vi "Mapping v10.0.0.vi"(5 "Simulate Spectra":bool, 7 "Simulate Drive":bool, 11 "Input Parameters":T7={"CCD3000 Connection"={"Comm Interface"=1, "BUS"=0, "Address"=5, "Com Port"=1}, "Drive Connection Settings"={"Objective GPIB-Port"=4, "Stage GPIB-Port"=4, "Drive Selector"=0, "Drive Velocity (V/s)"=5.0}, "ITC503 Current Values"={"ITC503 Heater"=0.0, "ITC503 Temperature"=0.0, "ITC503 P"=0.0, "ITC503 I"=0.0, "ITC503 D"=0.0, "ITC503 Setpoint"=0.0, "ITC503 Gradient"=0.0, "ITC503 Heater Auto"=FALSE, "ITC503 PID Auto"=FALSE}, "Wavelengths (nm)"=[], "Drive Current Values"={"Voltages"={"Drive X Voltage"=0.0, "Drive Y Voltage"=0.0, "Drive Z Voltage"=0.0}, "Position"={"Drive X Position"=0.0, "Drive Y Position"=0.0, "Drive Z Position"=0.0}}, "iHR Current Values"={"iHR 550 Front Entrance"=0.0, "iHR550 Side Exit"=0.0, "iHR550 Wavelength"=897.9988, "iHR550 Exit Mirror"=2, "iHR550 Grating"="1", "Grating Index"=1}, "Spectra Settings"={"Integration Time"=1.0, "Repetitions"=1, "Mapping Spectra"=TRUE}, "CCD3500 Temperature"=0.0} {"CCD3500 Temperature" min=10.0 max=160.0 step=0.1 format="%.1f"; "Spectra Settings"."Repetitions" min=1 max=100 step=1; "Spectra Settings"."Integration Time" min=0.5 max=6000.0 step=1.0 format="%.1f"; "iHR Current Values"."iHR550 Exit Mirror" items=["EntranceMirror", "ExitMirror", "Front", "Side"]; "Drive Current Values"."Position"."Drive Z Position" min=-273.0 max=300000.0 step=0.0001 format="%.1f"; "Drive Current Values"."Position"."Drive Y Position" min=-273.0 max=300000.0 step=0.0001 format="%.1f"; "Drive Current Values"."Position"."Drive X Position" min=-273.0 max=300000.0 step=0.0001 format="%.1f"; "Drive Current Values"."Voltages"."Drive Z Voltage" min=-273.0 max=300000.0 step=0.0001 format="%.1f"; "Drive Current Values"."Voltages"."Drive Y Voltage" min=-273.0 max=300000.0 step=0.0001 format="%.1f"; "Drive Current Values"."Voltages"."Drive X Voltage" min=-273.0 max=300000.0 step=0.0001 format="%.1f"; "ITC503 Current Values"."ITC503 Gradient" format="%.2f"; "ITC503 Current Values"."ITC503 Setpoint" min=-273.0 max=300000.0 step=0.0001 format="%.1f"; "ITC503 Current Values"."ITC503 I" format="%_1f"; "ITC503 Current Values"."ITC503 P" format="%_1f"; "ITC503 Current Values"."ITC503 Temperature" min=0.0 max=1645.0 step=1e-05 format="%.2f"; "ITC503 Current Values"."ITC503 Heater" min=0.0 max=100.0 step=0.01 scale=0.0..100.0; "Drive Connection Settings"."Drive Velocity (V/s)" min=10.0 max=160.0 step=0.1 format="%.1f"; "Drive Connection Settings"."Drive Selector" items=["Obj.", "Stage"]; "Drive Connection Settings"."Stage GPIB-Port" min=1 max=20 step=1 format="%#.0f"; "Drive Connection Settings"."Objective GPIB-Port" min=1 max=20 step=1 format="%#.0f"; "CCD3000 Connection"."Comm Interface" items=["RS 232", "GPIB"]}) -> ()   [LabVIEW 2010]
uses:
  ESA-C/TypeDefs/ESA-C Connection Settings.ctl
  TypeDefs/Mapping Spectra Params.ctl
  TypeDefs/Mapping Drive Params.ctl
  ESA-C/TypeDefs/ESA-C Set Positions.ctl
  ESA-C/TypeDefs/ESA-C Current Values.ctl
  iHR550/TypeDefs/iHR Current Values.ctl
  ITC503/TypeDefs/ITC503 Current Values.ctl
  drivers/Horiba Spectrum One 3000V/Lib/CCD_command.llb/Comm Params.ctl
  <vilib>/Utility/miscctls.llb/LVPointTypeDef.ctl
panel:
  in  "CCD3000 Current Rep.":string="0/0"
  in  "CCD3500V Connection":T8={"Comm Interface"=1, "BUS"=0, "Address"=5, "Com Port"=0}
  out "Live Data":dbl[][](array[numeric])
  in  "ITC503 Current Values":T3 {"ITC503 Gradient" format="%.2f"; "ITC503 Setpoint" min=-273.0 max=300000.0 step=0.0001 format="%.1f"; "ITC503 I" format="%_1f"; "ITC503 P" format="%_1f"; "ITC503 Temperature" min=0.0 max=1645.0 step=1e-05 format="%.2f"; "ITC503 Heater" min=0.0 max=100.0 step=0.01 scale=0.0..100.0}
  in  "iHR Current Values":T5={"iHR 550 Front Entrance"=0.0, "iHR550 Side Exit"=0.0, "iHR550 Wavelength"=897.9988, "iHR550 Exit Mirror"=2, "iHR550 Grating"="1", "Grating Index"=1} {"iHR550 Exit Mirror" items=["EntranceMirror", "ExitMirror", "Front", "Side"]}
  in  "CCD3500 Temperature":dbl caption="Temp. (°C)" min=10.0 max=160.0 step=0.1 format="%.1f"
  in  "Wavelengths (nm)":dbl[](array[numeric])
  in  "Spectra Params":T6={"Integration Time"=10.0, "Repetitions"=10, "Mapping Spectra"=TRUE} {"Repetitions" min=1 max=100 step=1; "Integration Time" min=0.5 max=6000.0 step=1.0 format="%.1f"}
  in  "Drive Settings":T2={"Objective GPIB-Port"=4, "Stage GPIB-Port"=4, "Drive Selector"=0, "Drive Velocity (V/s)"=5.0} {"Drive Velocity (V/s)" min=10.0 max=160.0 step=0.1 format="%.1f"; "Drive Selector" items=["Obj.", "Stage"]; "Stage GPIB-Port" min=1 max=20 step=1 format="%#.0f"; "Objective GPIB-Port" min=1 max=20 step=1 format="%#.0f"}
  out "Current Position":T4 {"Position"."Drive Z Position" min=-273.0 max=300000.0 step=0.0001 format="%.1f"; "Position"."Drive Y Position" min=-273.0 max=300000.0 step=0.0001 format="%.1f"; "Position"."Drive X Position" min=-273.0 max=300000.0 step=0.0001 format="%.1f"; "Voltages"."Drive Z Voltage" min=-273.0 max=300000.0 step=0.0001 format="%.1f"; "Voltages"."Drive Y Voltage" min=-273.0 max=300000.0 step=0.0001 format="%.1f"; "Voltages"."Drive X Voltage" min=-273.0 max=300000.0 step=0.0001 format="%.1f"}
  out "Target Position":T9={"Drive X Set"=10.0, "Drive Y Set"=10.0, "Drive Z Set"=10.0} {"Drive X Set" min=10.0 max=160.0 step=0.1 format="%.1f"; "Drive Z Set" min=10.0 max=160.0 step=0.1 format="%.1f"; "Drive Y Set" min=10.0 max=160.0 step=0.1 format="%.1f"}
  out "Progress":u8(slide) max=10 scale=0.0..100.0
  out "Objective Running":bool caption="Obj."
  out "CCD Running":bool caption="CCD"
  in  "Z Position":dbl caption="Z (µm)" min=0.0 max=100.0 step=0.1 format="%.1f"
  in  "Mapping Params":T10={"X Start Position"=0.0, "X Stop Position"=10.0, "Y Start Position"=0.0, "Y Stop Position"=10.0, "Step Size"=1.0} {"Step Size" min=0.1 max=30.0 step=0.1 format="%.1f"; "Y Stop Position" min=0.0 max=30.0 step=0.1 format="%.1f"; "Y Start Position" min=0.0 max=30.0 step=0.1 format="%.1f"; "X Stop Position" min=0.0 max=30.0 step=0.1 format="%.1f"; "X Start Position" min=0.0 max=30.0 step=0.1 format="%.1f"}
  in  "Exit":bool
  out "Measuring":bool
  in  "Start":bool
  # "Spectral"
  # "Spectral / Video Mapping"
  # "Parameters"
  # "GPIB"
  # "Status"
  # "Active"
  # "Target"
  # "Current"
  # "Mapping"
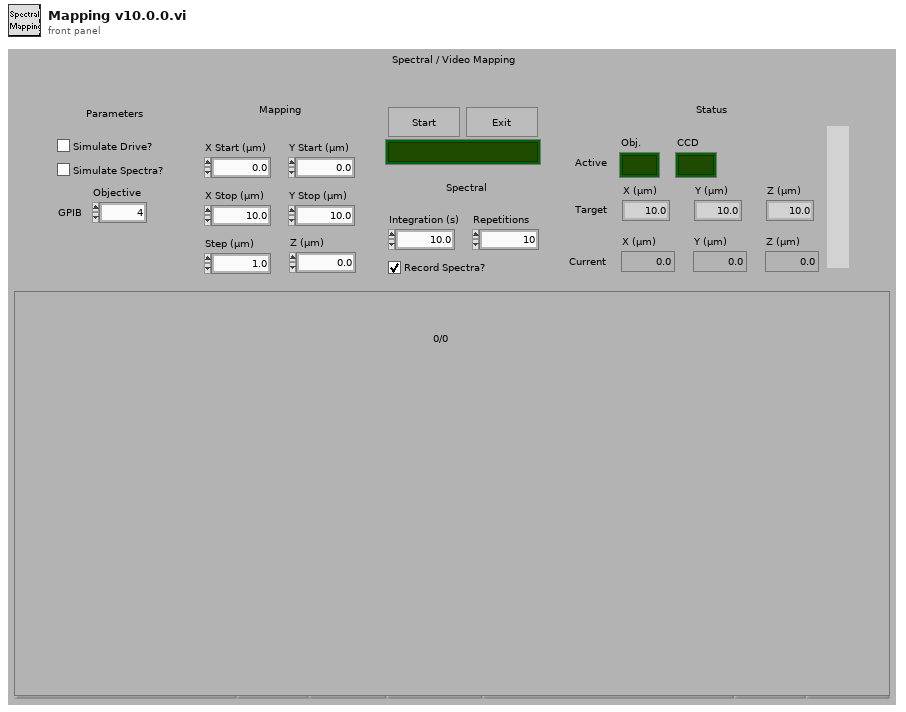
[diagram p1: front panel]
types:
  T1 = typedef "Comm Params.ctl" = cluster{"Comm Interface":u16, "BUS":i16, "Address":i16, "Com Port":i32}
  T2 = typedef "ESA-C Connection Settings.ctl" = cluster{"Objective GPIB-Port":i32, "Stage GPIB-Port":i32, "Drive Selector":u16, "Drive Velocity (V/s)":dbl}
  T3 = typedef "ITC503 Current Values.ctl" = cluster{"ITC503 Heater":dbl, "ITC503 Temperature":dbl, "ITC503 P":dbl, "ITC503 I":dbl, "ITC503 D":dbl, "ITC503 Setpoint":dbl, "ITC503 Gradient":dbl, "ITC503 Heater Auto":bool, "ITC503 PID Auto":bool}
  T4 = typedef "ESA-C Current Values.ctl" = cluster{"Voltages":cluster{"Drive X Voltage":dbl, "Drive Y Voltage":dbl, "Drive Z Voltage":dbl}, "Position":cluster{"Drive X Position":dbl, "Drive Y Position":dbl, "Drive Z Position":dbl}}
  T5 = typedef "iHR Current Values.ctl" = cluster{"iHR 550 Front Entrance":dbl, "iHR550 Side Exit":dbl, "iHR550 Wavelength":dbl, "iHR550 Exit Mirror":i32, "iHR550 Grating":string, "Grating Index":i32}
  T6 = typedef "Mapping Spectra Params.ctl" = cluster{"Integration Time":dbl, "Repetitions":u16, "Mapping Spectra":bool}
  T7 = cluster{"CCD3000 Connection":T1, "Drive Connection Settings":T2, "ITC503 Current Values":T3, "Wavelengths (nm)":dbl[], "Drive Current Values":T4, "iHR Current Values":T5, "Spectra Settings":T6, "CCD3500 Temperature":dbl}
  T8 = cluster{"Comm Interface":u16, "BUS":i16, "Address":i16, "Com Port":i32}
  T9 = typedef "ESA-C Set Positions.ctl" = cluster{"Drive X Set":dbl, "Drive Y Set":dbl, "Drive Z Set":dbl}
  T10 = typedef "Mapping Drive Params.ctl" = cluster{"X Start Position":dbl, "X Stop Position":dbl, "Y Start Position":dbl, "Y Stop Position":dbl, "Step Size":dbl}
  T11 = typedef "LVPointTypeDef.ctl" = cluster{"Horizontal":i16, "Vertical":i16}
  T12 = typedef "NPC3SG Set Positions.ctl" = cluster{"Drive X Set":dbl, "Drive Y Set":dbl, "Drive Z Set":dbl}
  T13 = cluster{"Intensities":dbl[], "Wavelengths":dbl[]}
  T14 = enum32{"invalid app kind", "Development System", "Run Time System", "Student Edition", "Embedded LabVIEW", "Evaluation", "Custom"}
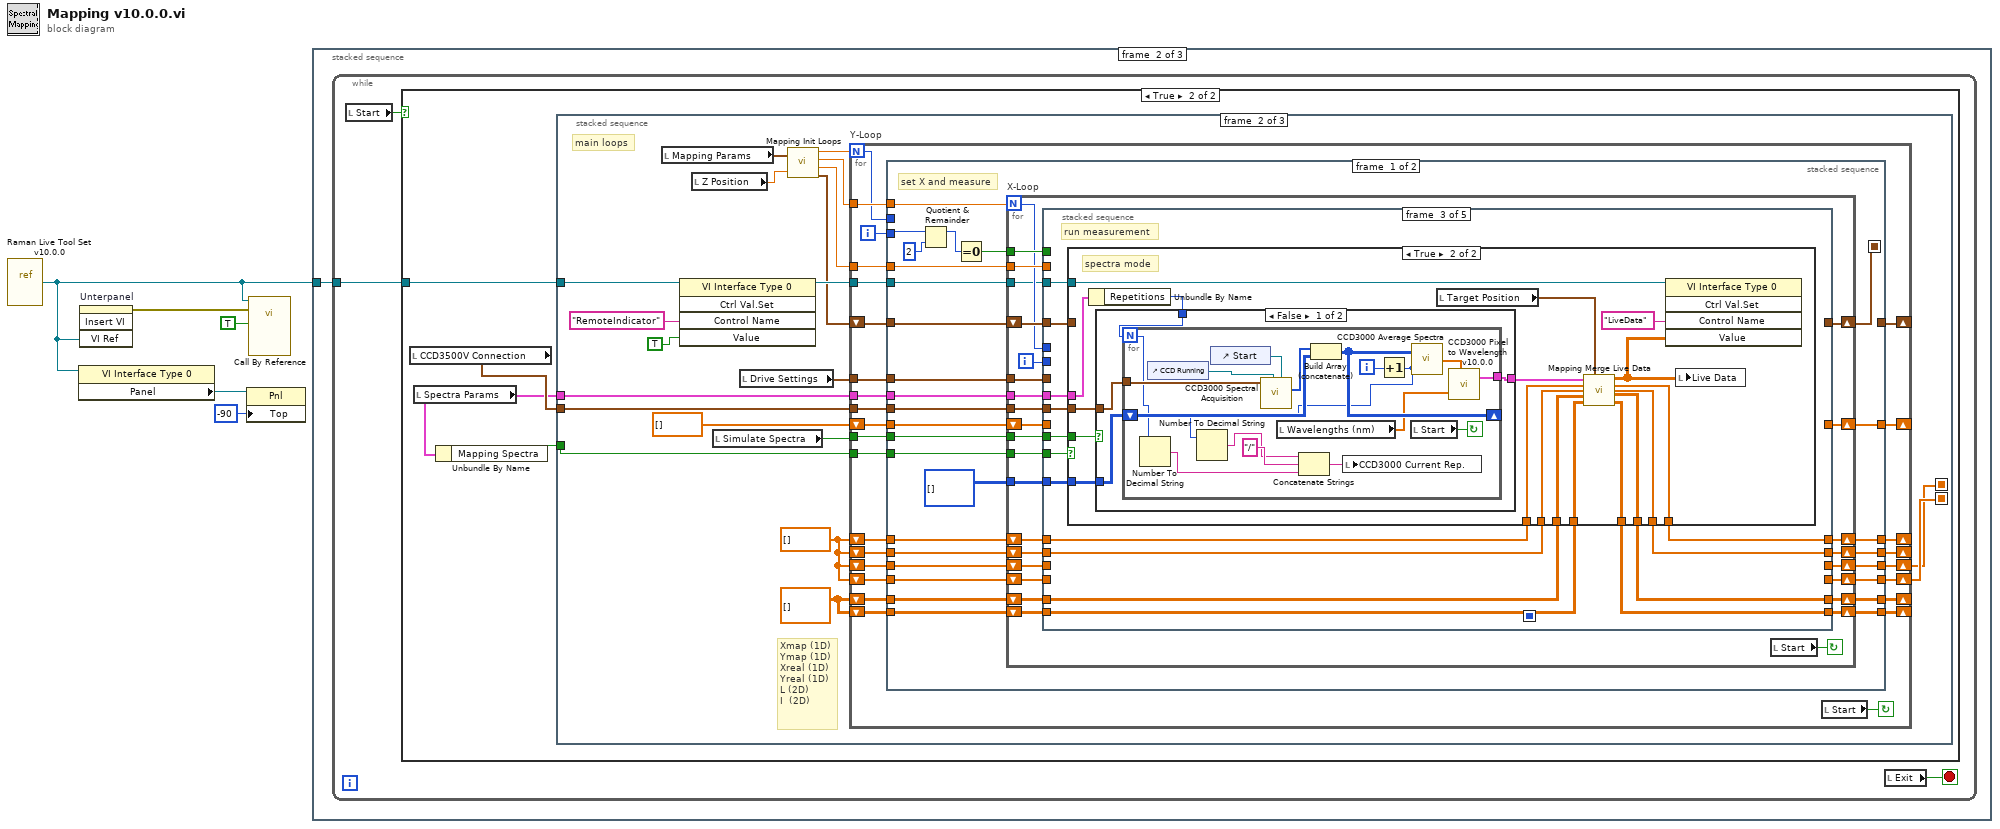
[diagram p0: block diagram]
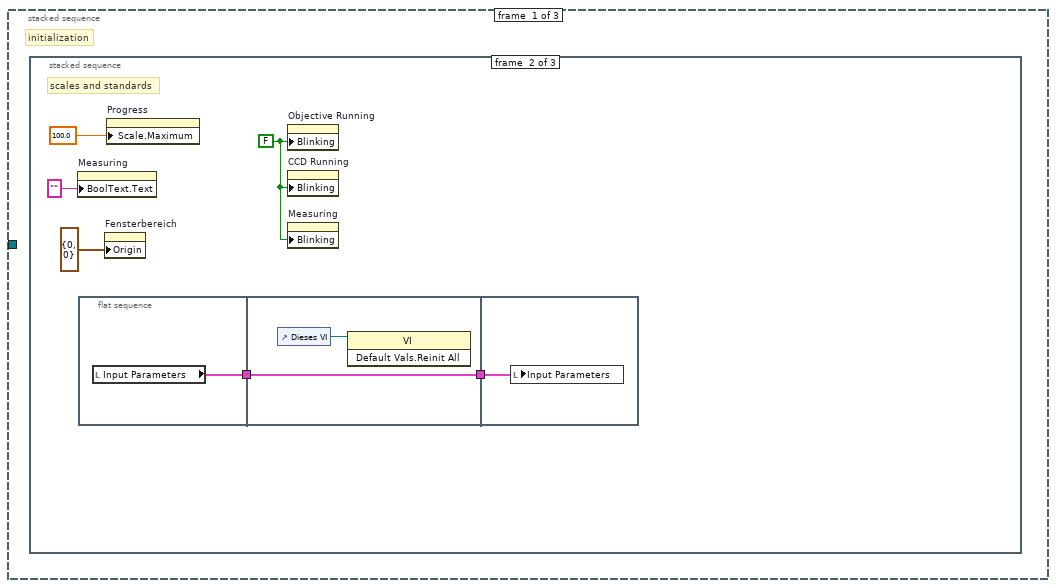
[diagram p2: hidden frame]
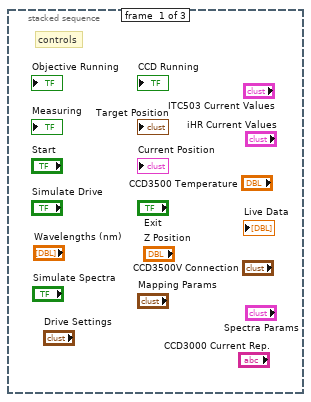
[diagram p3: hidden frame]
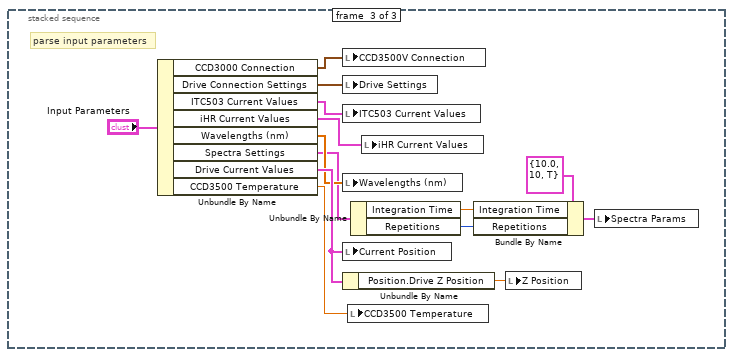
[diagram p4: hidden frame]
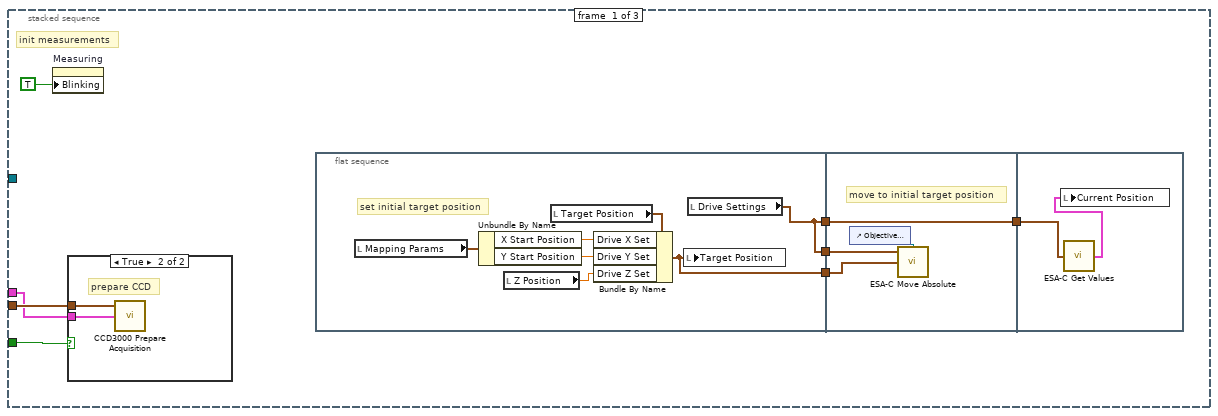
[diagram p6: hidden frame]
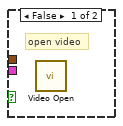
[diagram p7: hidden frame]
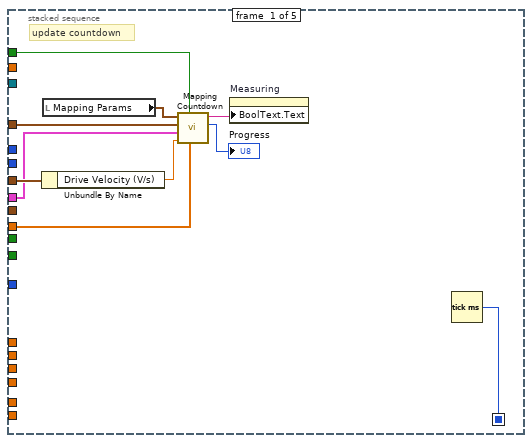
[diagram p8: hidden frame]
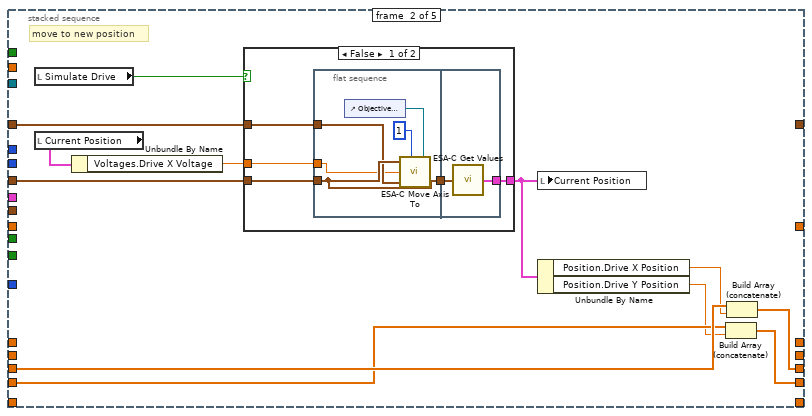
[diagram p9: hidden frame]
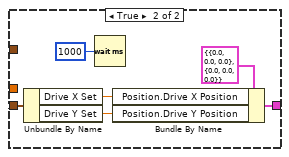
[diagram p10: hidden frame]
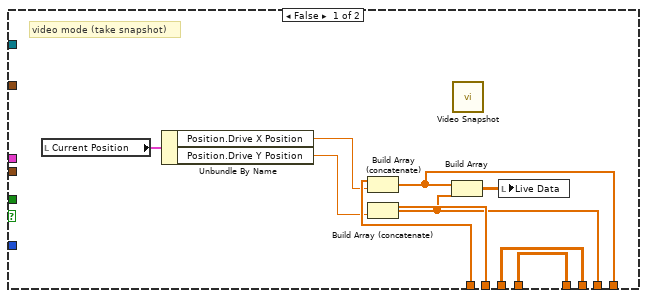
[diagram p11: hidden frame]
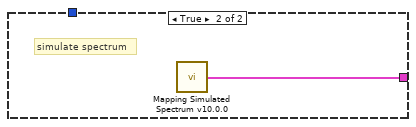
[diagram p12: hidden frame]
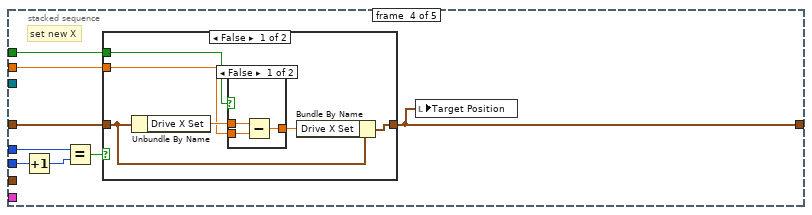
[diagram p13: hidden frame]
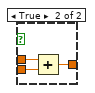
[diagram p14: hidden frame]
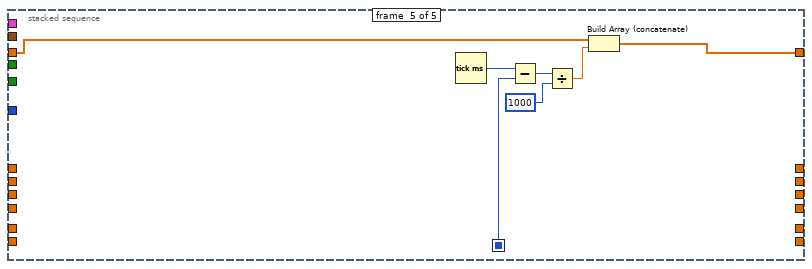
[diagram p16: hidden frame]
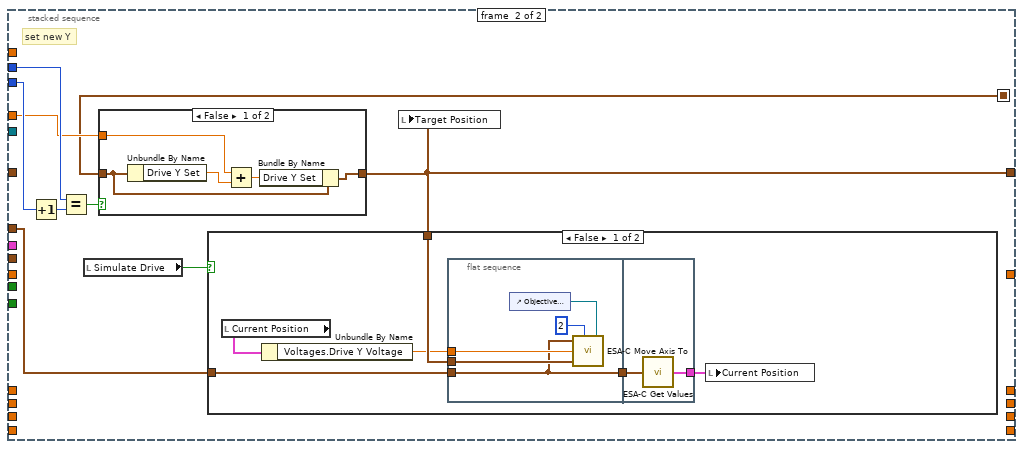
[diagram p17: hidden frame]
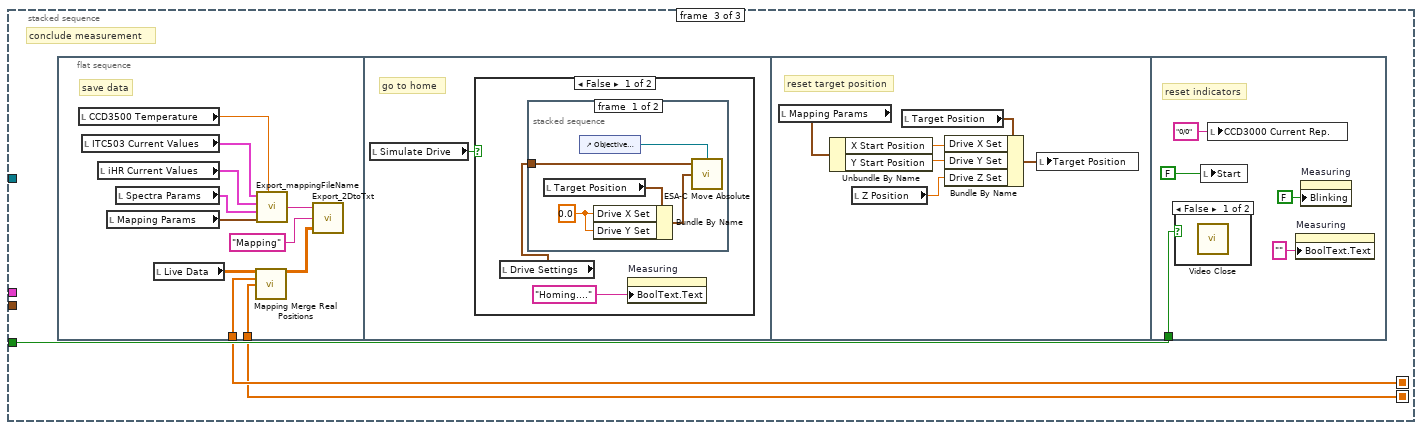
[diagram p20: hidden frame]
diagram:
  n1 = vi-ref "Raman Live Tool Set v10.0.0.vi"() -> (w3:refnum<vi>)
  n2 = property class="VI Interface Type 0"(reference=w3) -> ("Panel"=w2:refnum<vi>)  [unwired: 1 in, 2 out]
  n3 = invoke on="Unterpanel" class="Unterpanel" method="Insert VI"("VI Ref"=w3) -> (error out=w5:errorcluster)  [unwired: 3 in, 3 out]
  n4 = property class="Pnl"(reference=w2, "Top"=-90 ("Position:Oben")) -> ()  [unwired: 1 in, 2 out]
  n5 = call-by-ref "?"(reference=w3, error in=w5, "RemoteIndicator"=TRUE) -> ()  [unwired: 3 in, 2 out]
  n6 = stacked-sequence {
    tunnel: w3 -> [_ w30 w365]
    frame #0 {
      # "initialization"
      n7 = stacked-sequence {
        frame #0 {
          # "controls"
        }
        frame #1 {
          w9 = FALSE ("Blinkend")
          # "scales and standards"
          n8 = property on="Measuring" class="Bool (strict)"("BoolText.Text"="" ("Boolescher Text.Text")) -> ()  [unwired: 2 in, 2 out]
          n9 = flat-sequence {
            tunnel: [w12] -> w6
            tunnel: [w13] -> w7
            tunnel: w6 -> [w13]
            tunnel: w7 -> [w15]
            frame #0 {
              n10 = local read "Input Parameters"() -> (w12:T7)
            }
            frame #1 {
              n11 = control-ref of="Dieses VI"() -> (w14:refnum<vi>)
              n12 = invoke class="VI" method="Default Vals.Reinit All"(reference=w14) -> ()  [unwired: 2 in, 3 out]
            }
            frame #2 {
              n13 = local write "Input Parameters"(w15) -> ()
            }
          }
          n14 = property on="Fensterbereich" class="Pane"("Origin"=T11 {"Horizontal"=0, "Vertical"=0}) -> ()  [unwired: 2 in, 2 out]
          n15 = property on="Progress" class="Slide (strict)"("Scale.Maximum"=100.0 ("Skalierung.Bereich:Maximum")) -> ()  [unwired: 2 in, 2 out]
          n16 = property on="Objective Running" class="Bool (strict)"("Blinking"=w9) -> ()  [unwired: 2 in, 2 out]
          n17 = property on="CCD Running" class="Bool (strict)"("Blinking"=w9) -> ()  [unwired: 2 in, 2 out]
          n18 = property on="Measuring" class="Bool (strict)"("Blinking"=w9) -> ()  [unwired: 2 in, 2 out]
        }
        frame #2 {
          # "parse input parameters"
          n19 = Unbundle By Name("Input Parameters") -> ("CCD3000 Connection"=w25:T1, "Drive Connection Settings"=w26:T2, "ITC503 Current Values"=w28:T3, "iHR Current Values"=w16:T5, "Wavelengths (nm)"=w24:dbl[], "Spectra Settings"=w22:T6, "Drive Current Values"=w29:T4, "CCD3500 Temperature"=w17:dbl)
          n20 = local write "CCD3500V Connection"(w25) -> ()
          n21 = local write "Drive Settings"(w26) -> ()
          n22 = local write "ITC503 Current Values"(w28) -> ()
          n23 = local write "Wavelengths (nm)"(w24) -> ()
          n24 = local write "Current Position"(w29) -> ()
          n25 = Unbundle By Name(w29) -> ("Position.Drive Z Position"=w23:dbl)
          n26 = local write "CCD3500 Temperature"(w17) -> ()
          n27 = Unbundle By Name(w22) -> ("Integration Time"=w20:dbl, "Repetitions"=w19:u16)
          n28 = local write "iHR Current Values"(w16) -> ()
          n29 = Bundle By Name(cluster=T6 {"Integration Time"=10.0, "Repetitions"=10, "Mapping Spectra"=TRUE} ("Mapping Spectra Settings"), "Integration Time"=w20, "Repetitions"=w19) -> (w18:T6)
          n30 = local write "Z Position"(w23) -> ()
          n31 = local write "Spectra Params"(w18) -> ()
        }
      }
    }
    frame #1 {
      n32 = while {
        tunnel: w30 -> [w33]
        stop <- w32 stop-if-true
        n33 = local read "Start"() -> (w31:bool)
        n34 = case shown="True" w31 {
          tunnel: w33 -> [_ w37]
          frame False {
          }
          frame True {
            n35 = local read "CCD3500V Connection"() -> (w35:T8)
            n36 = local read "Spectra Params"() -> (w34:T6)
            n37 = Unbundle By Name(w34) -> ("Mapping Spectra"=w36:bool)
            n38 = stacked-sequence {
              seq-local: [_ w61 _] -> [_ _ w327]
              seq-local: [_ w62 _] -> [_ _ w326]
              tunnel: w37 -> [_ w72 _]
              tunnel: w36 -> [w44 w71 w328]
              tunnel: w34 -> [w42 w69 _]
              tunnel: w35 -> [w43 w68 _]
              frame #0 {
                # "init measurements"
                n39 = property on="Measuring" class="Bool (strict)"("Blinking"=TRUE ("Blinkend")) -> ()  [unwired: 2 in, 2 out]
                n40 = case shown="True" w44 {
                  tunnel: w43 -> [_ w60]
                  tunnel: w42 -> [_ w59]
                  frame False {
                    # "open video"
                    n41 = call "Video Open.vi"() -> ()  [unwired: 11 in, 1 out]
                  }
                  frame True {
                    # "prepare CCD"
                    n42 = call "CCD3000 Prepare Acquisition.vi"("Mapping Spectra Settings"=w59, "Comm Params"=w60) -> ()  [unwired: 4 in]
                  }
                }
                n43 = flat-sequence {
                  tunnel: [w47] -> w41
                  tunnel: [w46] -> w40
                  tunnel: [w46] -> w38
                  tunnel: w41 -> [w56]
                  tunnel: w40 -> [w55]
                  tunnel: [w54] -> w39
                  tunnel: w38 -> [w54]
                  tunnel: w39 -> [w58]
                  frame #0 {
                    # "set initial target position"
                    n44 = local read "Mapping Params"() -> (w52:T10)
                    n45 = Unbundle By Name(w52) -> ("X Start Position"=w50:dbl, "Y Start Position"=w49:dbl)
                    n46 = local read "Z Position"() -> (w48:dbl)
                    n47 = local read "Target Position"() -> (w51:T9)
                    n48 = Bundle By Name(cluster=w51, "Drive X Set"=w50, "Drive Y Set"=w49, "Drive Z Set"=w48) -> (w47:T9)
                    n49 = local write "Target Position"(w47) -> ()
                    n50 = local read "Drive Settings"() -> (w46:T2)
                  }
                  frame #1 {
                    # "move to initial target position"
                    n51 = control-ref of="Objective Running"() -> (w53:refnum<vi>)
                    n52 = call "ESA-C Move Absolute.vi"("Running"=w53, "Drive New Abs. Positions"=w56, "Drive Connection Settings"=w55) -> ()  [unwired: 2 in]
                  }
                  frame #2 {
                    n53 = call "ESA-C Get Values.vi"("Drive Connection Settings"=w58) -> ("Drive Current Values"=w57:T4)
                    n54 = local write "Current Position"(w57) -> ()
                  }
                }
              }
              frame #1 {
                w80 = dbl[][] []
                w63 = dbl[] []
                # "main loops"
                # "Xmap (1D)\nYmap (1D)\nXreal (1D)\nYreal (1D)\nL (2D)\nI  (2D)"
                n55 = local read "Mapping Params"() -> (w66:T10)
                n56 = invoke class="VI Interface Type 0" method="Ctrl Val.Set"(reference=w72, "Control Name"="RemoteIndicator" ("Elementname"), "Value"=TRUE) -> (reference out=w74:refnum<vi>)  [unwired: 2 in, 4 out]
                n57 = local read "Z Position"() -> (w65:dbl)
                n58 = local read "Simulate Spectra"() -> (w64:bool)
                n59 = local read "Drive Settings"() -> (w67:T2)
                n60 = call "Mapping Init Loops.vi"("Z Position"=w65, "Mapping Params"=w66) -> ("Start Positions"=w73:T12, "Step Size"=w75:dbl, "X Steps"=w76:dbl, "Y Steps"=w77:dbl)
                n61 = for "Y-Loop" {
                  N: w77 -> [w93]
                  tunnel: w76 -> [w106]
                  tunnel: w75 -> [w105]
                  shift-right: [w91] -> _
                  shift-left: w73 -> [w92]
                  shift-right: [w97] -> _
                  shift-left: w80 -> [w101]
                  shift-right: [w98] -> _
                  shift-left: w80 -> [w102]
                  shift-right: [w100] -> _
                  shift-left: w63 -> [w104]
                  shift-right: [w99] -> _
                  shift-left: w63 -> [w103]
                  tunnel: w74 -> [w95]
                  tunnel: w64 -> [w94]
                  tunnel: w67 -> [w90]
                  tunnel: w71 -> [w89]
                  tunnel: w69 -> [w88]
                  shift-right: [w86] -> _
                  shift-left: dbl[] [] -> [w87]
                  tunnel: w68 -> [w85]
                  shift-right: [w82] -> w62
                  shift-left: w63 -> [w83]
                  shift-right: [w81] -> w61
                  shift-left: w63 -> [w84]
                  i -> [w96]
                  stop <- w107 continue-if-true
                  n62 = stacked-sequence {
                    seq-local: [w120 _] -> [_ w301]
                    tunnel: w106 -> [w136 _]
                    tunnel: w105 -> [w135 w302]
                    tunnel: w104 -> [w134 _]
                    tunnel: w103 -> [w133 _]
                    tunnel: w102 -> [w132 _]
                    tunnel: w101 -> [w131 _]
                    tunnel: [w130 _] -> w100
                    tunnel: [w129 _] -> w99
                    tunnel: [w128 _] -> w98
                    tunnel: [w127 _] -> w97
                    tunnel: w96 -> [w124 w306]
                    tunnel: w95 -> [w122 _]
                    tunnel: w94 -> [w121 _]
                    tunnel: w93 -> [_ w304]
                    tunnel: w92 -> [w119 _]
                    tunnel: [_ w299] -> w91
                    tunnel: w90 -> [w118 w300]
                    tunnel: w89 -> [w117 _]
                    tunnel: w88 -> [w116 _]
                    tunnel: w87 -> [w115 _]
                    tunnel: [w114 _] -> w86
                    tunnel: w85 -> [w113 _]
                    tunnel: w84 -> [w111 _]
                    tunnel: w83 -> [w110 _]
                    tunnel: [w109 _] -> w82
                    tunnel: [w108 _] -> w81
                    frame #0 {
                      # "set X and measure"
                      n63 = Quotient & Remainder(x=w124, y=2) -> (x-y*floor(x/y)=w125:i32)  [unwired: 1 out]
                      n64 = Equal To 0?(x=w125) -> (x = 0?=w123:bool)
                      n65 = for "X-Loop" {
                        N: w136 -> [w150]
                        tunnel: w135 -> [w162]
                        shift-right: [w161] -> w120
                        shift-left: w119 -> [w163]
                        shift-right: [w156] -> w130
                        shift-left: w134 -> [w160]
                        shift-right: [w155] -> w129
                        shift-left: w133 -> [w159]
                        shift-right: [w153] -> w128
                        shift-left: w132 -> [w158]
                        shift-right: [w154] -> w127
                        shift-left: w131 -> [w157]
                        tunnel: w123 -> [w152]
                        tunnel: w122 -> [w149]
                        tunnel: w121 -> [w148]
                        tunnel: w118 -> [w147]
                        tunnel: w117 -> [w146]
                        tunnel: w116 -> [w145]
                        shift-right: [w144] -> w114
                        shift-left: w115 -> [w143]
                        tunnel: w113 -> [w142]
                        tunnel: u16[][] [] -> [w141]
                        shift-right: [w137] -> w108
                        shift-left: w111 -> [w140]
                        shift-right: [w138] -> w109
                        shift-left: w110 -> [w139]
                        i -> [w151]
                        stop <- w164 continue-if-true
                        n66 = stacked-sequence {
                          seq-local: [w165 _ _ _ _] -> [_ _ _ _ w294]
                          tunnel: w163 -> [w170 w186 w219 w273 _]
                          tunnel: w162 -> [_ _ _ w271 _]
                          tunnel: [_ _ _ w270 _] -> w161
                          tunnel: w160 -> [_ _ w218 _ _]
                          tunnel: w159 -> [_ _ w217 _ _]
                          tunnel: w158 -> [_ _ w215 _ _]
                          tunnel: w157 -> [_ _ w216 _ _]
                          tunnel: [_ _ w214 _ _] -> w156
                          tunnel: [_ _ w213 _ _] -> w155
                          tunnel: [_ _ w212 _ _] -> w154
                          tunnel: [_ _ w211 _ _] -> w153
                          tunnel: w152 -> [w171 _ _ w272 _]
                          tunnel: w151 -> [_ _ _ w277 _]
                          tunnel: w150 -> [_ _ _ w274 _]
                          tunnel: w149 -> [_ _ w210 _ _]
                          tunnel: w148 -> [_ _ w209 _ _]
                          tunnel: w147 -> [w168 w184 _ _ _]
                          tunnel: w146 -> [_ _ w208 _ _]
                          tunnel: w145 -> [w167 _ w206 _ _]
                          tunnel: [_ _ _ _ w291] -> w144
                          tunnel: w143 -> [w166 _ _ _ w293]
                          tunnel: w142 -> [_ _ w207 _ _]
                          tunnel: w141 -> [_ _ w205 _ _]
                          tunnel: w140 -> [_ w180 _ _ _]
                          tunnel: w139 -> [_ w179 _ _ _]
                          tunnel: [_ w176 _ _ _] -> w138
                          tunnel: [_ w175 _ _ _] -> w137
                          frame #0 {
                            # "update countdown"
                            n67 = Unbundle By Name(w168) -> ("Drive Velocity (V/s)"=w169:dbl)
                            n68 = local read "Mapping Params"() -> (w174:T10)
                            n69 = call "Mapping Countdown.vi"("Execution Times (s)"=w166, "Forward?"=w171, "Drive Velocity"=w169, "Mapping Spectra Settings"=w167, "Drive New Abs. Positions"=w170, "Mapping Drive Parameters"=w174) -> ("Progress"=→"Progress":i16, "Time String"=w172:string)  [unwired: 4 in]
                            n70 = property on="Measuring" class="Bool (strict)"("BoolText.Text"=w172) -> ()  [unwired: 2 in, 2 out]
                            n71 = Tick Count (ms)() -> (millisecond timer value=w165:u32)
                          }
                          frame #1 {
                            # "move to new position"
                            n72 = local read "Simulate Drive"() -> (w185:bool)
                            n73 = local read "Current Position"() -> (w183:T4)
                            n74 = Unbundle By Name(w183) -> ("Voltages.Drive X Voltage"=w182:dbl)
                            n75 = case shown="False" w185 {
                              tunnel: w186 -> [w190 w203]
                              tunnel: [w189 w200] -> w181
                              tunnel: w184 -> [w188 _]
                              tunnel: w182 -> [w187 _]
                              frame False {
                                n76 = flat-sequence {
                                tunnel: w190 -> [w195]
                                tunnel: [w196] -> w191
                                tunnel: w188 -> [w196]
                                tunnel: w187 -> [w192]
                                tunnel: w191 -> [w198]
                                tunnel: [w197] -> w189
                                frame #0 {
                                n77 = control-ref of="Objective Running"() -> (w193:refnum<vi>)
                                n78 = call "ESA-C Move Axis To.vi"("Drive Connection Settings"=w196, "Axis"=1, "Current Voltage (V)"=w192, "Drive New Abs. Positions"=w195, "Running"=w193) -> ()  [unwired: 2 in]
                                }
                                frame #1 {
                                n79 = call "ESA-C Get Values.vi"("Drive Connection Settings"=w198) -> ("Drive Current Values"=w197:T4)
                                }
                                }
                              }
                              frame True {
                                n80 = Unbundle By Name(w203) -> ("Drive X Set"=w204:dbl, "Drive Y Set"=w201:dbl)
                                n81 = Wait (ms)(milliseconds to wait=u32 1000 ("Zu wartende ms")) -> ()  [unwired: 1 out]
                                n82 = Bundle By Name(cluster=T4 {"Voltages"={"Drive X Voltage"=0.0, "Drive Y Voltage"=0.0, "Drive Z Voltage"=0.0}, "Position"={"Drive X Position"=0.0, "Drive Y Position"=0.0, "Drive Z Position"=0.0}} ("Drive Current Values"), "Position.Drive X Position"=w204, "Position.Drive Y Position"=w201) -> (w200:T4)
                              }
                            }
                            n83 = local write "Current Position"(w181) -> ()
                            n84 = Unbundle By Name(w181) -> ("Position.Drive X Position"=w178:dbl, "Position.Drive Y Position"=w177:dbl)
                            n85 = Build Array (concatenate)(w179, w177) -> (w176:dbl[])
                            n86 = Build Array (concatenate)(w180, w178) -> (w175:dbl[])
                          }
                          frame #2 {
                            # "run measurement"
                            n87 = case shown="True" w208 {
                              tunnel: w219 -> [_ _]
                              tunnel: w218 -> [w226 w244]
                              tunnel: w217 -> [w225 w243]
                              tunnel: w216 -> [w228 w241]
                              tunnel: w215 -> [w229 w242]
                              tunnel: [w223 w238] -> w214
                              tunnel: [w224 w237] -> w213
                              tunnel: [w228 w240] -> w212
                              tunnel: [w229 w239] -> w211
                              tunnel: w210 -> [_ w246]
                              tunnel: w209 -> [_ w245]
                              tunnel: w207 -> [_ w233]
                              tunnel: w206 -> [_ w232]
                              tunnel: w205 -> [_ w230]
                              frame False {
                                # "video mode (take snapshot)"
                                n88 = local read "Current Position"() -> (w227:T4)
                                n89 = Unbundle By Name(w227) -> ("Position.Drive X Position"=w222:dbl, "Position.Drive Y Position"=w221:dbl)
                                n90 = Build Array (concatenate)(w226, w222) -> (w223:dbl[])
                                n91 = Build Array (concatenate)(w225, w221) -> (w224:dbl[])
                                n92 = Build Array(w223, w224) -> (w220:dbl[][])
                                n93 = call "Video Snapshot.vi"() -> ()  [unwired: 11 in, 1 out]
                                n94 = local write "Live Data"(w220) -> ()
                              }
                              frame True {
                                # "spectra mode"
                                n95 = Unbundle By Name(w232) -> ("Repetitions"=w231:u16)
                                n96 = case shown="False" w245 {
                                tunnel: [w250 w269] -> w236
                                tunnel: w233 -> [w251 _]
                                tunnel: w231 -> [w249 _]
                                tunnel: w230 -> [w248 _]
                                frame False {
                                n97 = for {
                                N: w249 -> [w253]
                                shift-right: [w265] -> _
                                shift-left: w248 -> [w266]
                                tunnel: [w263] -> w250
                                tunnel: w251 -> [w261]
                                i -> [w268]
                                stop <- w260 continue-if-true
                                n98 = Number To Decimal String(number=w253) -> (decimal integer string=w256:string)  [unwired: 1 in]
                                n99 = control-ref of="CCD Running"() -> (w259:refnum<vi>)
                                n100 = control-ref of="Start"() -> (w258:refnum<vi>)
                                n101 = call "CCD3000 Spectral Acquisition.vi"("Acquire"=w258, "Running"=w259, "Comm Params"=w261) -> ("Raw-Spectrum"=w267:u16[])  [unwired: 6 in, 2 out]
                                n102 = local read "Wavelengths (nm)"() -> (w262:dbl[])
                                n103 = Build Array (concatenate)(w267, w266) -> (w265:u16[][])
                                n104 = Increment(x=w268) -> (x+1=w252:i32)
                                n105 = Number To Decimal String(number=w252) -> (decimal integer string=w255:string)  [unwired: 1 in]
                                n106 = Concatenate Strings(w255, "/" ("string"), w256) -> (w254:string)
                                n107 = local write "CCD3000 Current Rep."(w254) -> ()
                                n108 = local read "Start"() -> (w260:bool)
                                n109 = call "CCD3000 Average Spectra.vi"("Repetitions"=w252, "Raw Spectra"=w265) -> ("Raw Spectrum"=w264:dbl[])
                                n110 = call "CCD3000 Pixel to Wavelength v10.0.0.vi"("Wavelengths (nm)"=w262, "Raw Spectrum"=w264) -> ("Spectrum-Cluster"=w263:T13)  [unwired: 1 out]
                                }
                                }
                                frame True {
                                # "simulate spectrum"
                                n111 = call "Mapping Simulated Spectrum v10.0.0.vi"() -> ("Simulated Spectrum"=w269:cluster{i32[], dbl[]})
                                }
                                }
                                n112 = local read "Target Position"() -> (w235:T9)
                                n113 = call "Mapping Merge Live Data.vi"("New Spectrum"=w236, "Target Position"=w235, "X in (1D)"=w244, "Y in (1D)"=w243, "L in (2D)"=w242, "I in (2D)"=w241) -> ("Live Data"=w234:dbl[][], "X out (1D)"=w238:dbl[], "Y out (1D)"=w237:dbl[], "L out (2D)"=w239:dbl[][], "I out (2D)"=w240:dbl[][])  [unwired: 5 in]
                                n114 = invoke class="VI Interface Type 0" method="Ctrl Val.Set"(reference=w246, "Control Name"="LiveData" ("Elementname"), "Value"=w234) -> ()  [unwired: 2 in, 5 out]
                                n115 = local write "Live Data"(w234) -> ()
                              }
                            }
                          }
                          frame #3 {
                            # "set new X"
                            n116 = Increment(x=w277) -> (x+1=w276:i32)
                            n117 = Equal?(x=w274, y=w276) -> (x = y?=w275:bool)
                            n118 = case shown="False" w275 {
                              tunnel: w273 -> [w281 w290]
                              tunnel: [w280 w290] -> w270
                              tunnel: w272 -> [w279 _]
                              tunnel: w271 -> [w278 _]
                              frame False {
                                n119 = Unbundle By Name(w281) -> ("Drive X Set"=w282:dbl)
                                n120 = case shown="False" w279 {
                                tunnel: w282 -> [w286 w288]
                                tunnel: [w285 w289] -> w283
                                tunnel: w278 -> [w284 w287]
                                frame False {
                                n121 = Subtract(x=w286, y=w284) -> (x-y=w285:dbl)
                                }
                                frame True {
                                n122 = Add(x=w288, y=w287) -> (x+y=w289:dbl)
                                }
                                }
                                n123 = Bundle By Name(cluster=w281, "Drive X Set"=w283) -> (w280:T12)
                              }
                              frame True {
                              }
                            }
                            n124 = local write "Target Position"(w270) -> ()
                          }
                          frame #4 {
                            n125 = Tick Count (ms)() -> (millisecond timer value=w295:u32)
                            n126 = Subtract(x=w295, y=w294) -> (x-y=w297:u32)
                            n127 = Divide(x=w297, y=u32 1000) -> (x/y=w292:dbl)
                            n128 = Build Array (concatenate)(w293, w292) -> (w291:dbl[])
                          }
                        }
                        n129 = local read "Start"() -> (w164:bool)
                      }
                    }
                    frame #1 {
                      # "set new Y"
                      n130 = Increment(x=w306) -> (x+1=w305:i32)
                      n131 = Equal?(x=w304, y=w305) -> (x = y?=w303:bool)
                      n132 = local read "Simulate Drive"() -> (w298:bool)
                      n133 = case shown="False" w303 {
                        tunnel: w301 -> [w324 w325]
                        tunnel: [w323 w325] -> w299
                        tunnel: w302 -> [w320 _]
                        frame False {
                          n134 = Unbundle By Name(w324) -> ("Drive Y Set"=w321:dbl)
                          n135 = Add(x=w320, y=w321) -> (x+y=w322:dbl)
                          n136 = Bundle By Name(cluster=w324, "Drive Y Set"=w322) -> (w323:T12)
                        }
                        frame True {
                        }
                      }
                      n137 = case shown="False" w298 {
                        tunnel: w300 -> [w310 _]
                        tunnel: w299 -> [w309 _]
                        frame False {
                          n138 = local read "Current Position"() -> (w308:T4)
                          n139 = Unbundle By Name(w308) -> ("Voltages.Drive Y Voltage"=w307:dbl)
                          n140 = flat-sequence {
                            tunnel: w310 -> [w313]
                            tunnel: w309 -> [w314]
                            tunnel: w307 -> [w315]
                            tunnel: [w313] -> w312
                            tunnel: [w319] -> w311
                            tunnel: w312 -> [w318]
                            frame #0 {
                              n141 = control-ref of="Objective Running"() -> (w317:refnum<vi>)
                              n142 = call "ESA-C Move Axis To.vi"("Drive Connection Settings"=w313, "Axis"=2, "Current Voltage (V)"=w315, "Drive New Abs. Positions"=w314, "Running"=w317) -> ()  [unwired: 2 in]
                            }
                            frame #1 {
                              n143 = call "ESA-C Get Values.vi"("Drive Connection Settings"=w318) -> ("Drive Current Values"=w319:T4)
                            }
                          }
                          n144 = local write "Current Position"(w311) -> ()
                        }
                        frame True {
                        }
                      }
                      n145 = local write "Target Position"(w299) -> ()
                    }
                  }
                  n146 = local read "Start"() -> (w107:bool)
                }
              }
              frame #2 {
                # "conclude measurement"
                n147 = flat-sequence {
                  tunnel: w327 -> [w330]
                  tunnel: w326 -> [w329]
                  tunnel: w328 -> [w357]
                  frame #0 {
                    # "save data"
                    n148 = local read "CCD3500 Temperature"() -> (w337:dbl)
                    n149 = local read "ITC503 Current Values"() -> (w339:T3)
                    n150 = local read "iHR Current Values"() -> (w338:T5)
                    n151 = local read "Mapping Params"() -> (w333:T10)
                    n152 = local read "Spectra Params"() -> (w334:T6)
                    n153 = local read "Live Data"() -> (w332:dbl[][])
                    n154 = call "Mapping Merge Real Positions.vi"("Live Data In"=w332, "X in (1D)"=w330, "Y in (1D)"=w329) -> ("Live Data Out"=w331:dbl[][])  [unwired: 12 in]
                    n155 = call "Export_mappingFileName.vi"("ITC503 Current Values"=w339, "iHR Current Values"=w338, "Spectra Settings"=w334, "Mapping Parameters"=w333, "CCD3500 Temperature"=w337) -> ("Filename"=w335:string)
                    n156 = call "Export_2DtoTxt.vi"("Data (2D)"=w331, "Export Type"="Mapping", "Filename"=w335) -> ()  [unwired: 3 in]
                  }
                  frame #1 {
                    # "go to home"
                    n157 = local read "Simulate Drive"() -> (w340:bool)
                    n158 = case shown="False" w340 {
                      frame False {
                        n159 = local read "Drive Settings"() -> (w341:T2)
                        n160 = stacked-sequence {
                          tunnel: w341 -> [w343 w349]
                          frame #0 {
                            w346 = 0.0 ("Drive Y Set")
                            n161 = local read "Target Position"() -> (w345:T9)
                            n162 = control-ref of="Objective Running"() -> (w344:refnum<vi>)
                            n163 = Bundle By Name(cluster=w345, "Drive X Set"=w346, "Drive Y Set"=w346) -> (w347:T9)
                            n164 = call "ESA-C Move Absolute.vi"("Running"=w344, "Drive New Abs. Positions"=w347, "Drive Connection Settings"=w343) -> ()  [unwired: 2 in]
                          }
                          frame #1 {
                            n165 = call "ESA-C Get Values.vi"("Drive Connection Settings"=w349) -> ("Drive Current Values"=w348:T4)
                            n166 = local write "Current Position"(w348) -> ()
                          }
                        }
                        n167 = property on="Measuring" class="Bool (strict)"("BoolText.Text"="Homing...." ("Boolescher Text.Text")) -> ()  [unwired: 2 in, 2 out]
                      }
                      frame True {
                      }
                    }
                  }
                  frame #2 {
                    # "reset target position"
                    n168 = local read "Mapping Params"() -> (w350:T10)
                    n169 = Unbundle By Name(w350) -> ("X Start Position"=w353:dbl, "Y Start Position"=w352:dbl)
                    n170 = local read "Z Position"() -> (w351:dbl)
                    n171 = local read "Target Position"() -> (w355:T9)
                    n172 = Bundle By Name(cluster=w355, "Drive X Set"=w353, "Drive Y Set"=w352, "Drive Z Set"=w351) -> (w354:T9)
                    n173 = local write "Target Position"(w354) -> ()
                  }
                  frame #3 {
                    # "reset indicators"
                    n174 = case shown="False" w357 {
                      frame False {
                        n175 = call "Video Close.vi"() -> ()  [unwired: 11 in, 1 out]
                      }
                      frame True {
                      }
                    }
                    n176 = local write "Start"(FALSE ("Start")) -> ()
                    n177 = local write "CCD3000 Current Rep."("0/0" ("CCD3000 Current Rep.")) -> ()
                    n178 = property on="Measuring" class="Bool (strict)"("BoolText.Text"="" ("Boolescher Text.Text")) -> ()  [unwired: 2 in, 2 out]
                    n179 = property on="Measuring" class="Bool (strict)"("Blinking"=FALSE ("Measuring")) -> ()  [unwired: 2 in, 2 out]
                  }
                }
              }
            }
          }
        }
        n180 = local read "Exit"() -> (w32:bool)
      }
    }
    frame #2 {
      # "reset and close"
      n181 = control-ref of="Dieses VI"() -> (w364:refnum<vi>)
      n182 = invoke class="VI Interface Type 0" method="Ctrl Val.Set"(reference=w365, "Control Name"="Exit" ("Elementname"), "Value"=TRUE) -> ()  [unwired: 2 in, 5 out]
      n183 = invoke class="VI" method="Default Vals.Reinit All"(reference=w364) -> (reference out=w362:refnum<vi>)  [unwired: 2 in, 2 out]
      n184 = property on="Measuring" class="Bool (strict)"("BoolText.Text"="" ("Boolescher Text.Text")) -> ()  [unwired: 2 in, 2 out]
      n185 = property class="App"() -> ("App.Kind"=w363:T14)  [unwired: 2 in, 2 out]
      n186 = case shown="\"Development System\"" w363 {
        tunnel: w362 -> [w368 _]
        frame "invalid app kind", Default {
          n187 = invoke on="Invoke Node" class="VI" method="FP.Close"(reference=w368) -> ()  [unwired: 2 in, 3 out]
        }
        frame "Development System" {
        }
      }
    }
  }
